vi "Counts_Freq and Temperature to Range.vi"(4 "Atm. Pressure (pascals)":dbl=101325.0, 6 "Oscillator freq":i32, 8 "Humidity (%)":dbl=60.0 format="%_4g", 9 "Range Counts":i32, 10 "Range":dbl, 11 "All Temps":dbl[](array[numeric])) -> (2 "Cramer Range (m)":dbl, 3 "Range (m)":dbl)   [LabVIEW 2019, in "Analysis.lvlib"]
uses:
  Analysis.lvlib
panel:
  # "101325"
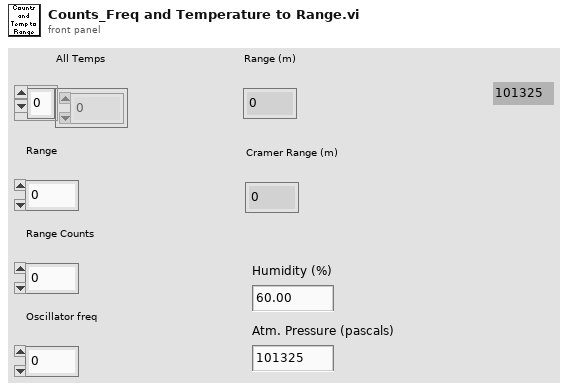
[diagram p1: front panel]
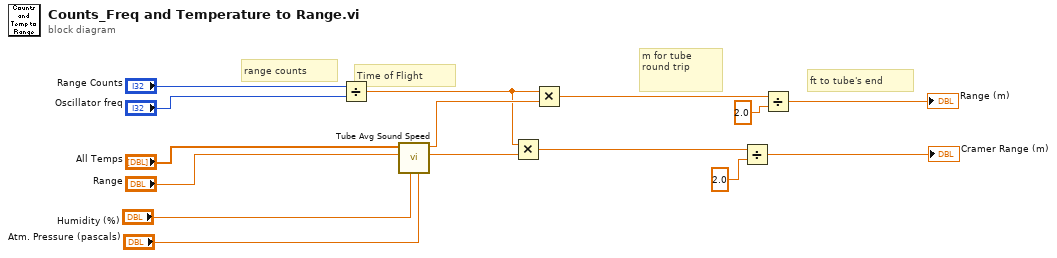
[diagram p0: block diagram]
diagram:
  # "ft to tube's end"
  # "m for tube \nround trip"
  # "Time of Flight"
  # "range counts"
  n1 = Divide(x="Range Counts", y="Oscillator freq") -> (x/y=w4:dbl)
  n2 = call "Tube Avg Sound Speed.vi"("Atm. Pressure (pascals)"="Atm. Pressure (pascals)", "Humidity (%)"="Humidity (%)", "Range"="Range", "All Temps"="All Temps") -> ("Cramer Speed of Sound in Tube Length at Tc"=w3:dbl, "Speed of Sound in Tube Length at Tc"=w13:dbl)  [unwired: 5 in, 1 out]
  n3 = Multiply(x=w4, y=w3) -> (x*y=w7:dbl)
  n4 = Multiply(x=w4, y=w13) -> (x*y=w8:dbl)
  n5 = Divide(x=w7, y=2.0) -> (x/y=→"Cramer Range (m)":dbl)
  n6 = Divide(x=w8, y=2.0) -> (x/y=→"Range (m)":dbl)
